vi "Get Errno Description.vi"(8 "error in":errorcluster, 11 "errnum":i32) -> (0 "error out":errorcluster, 3 "Description":string)   [LabVIEW 2018, in "PCANBasic.lvlib" / "epoll.lvclass"]
uses:
  epoll.lvclass
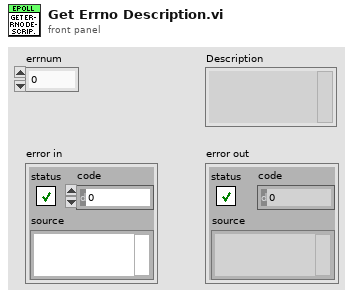
[diagram p1: front panel]
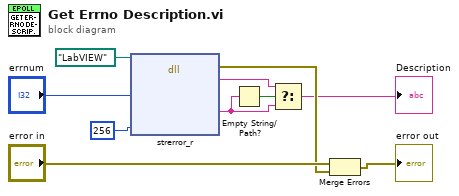
[diagram p0: block diagram]
diagram:
  n1 = dll-call lib="LabVIEW" fn="strerror_r"(path in=path "LabVIEW", "errnum"="errnum", "string_len"=256) -> (error out=w4:errorcluster, "return"=w6:string, "string"=w7:string)  [unwired: 5 in, 1 out]
  n2 = Empty String/Path?(string/path=w7) -> (empty?=w8:bool)
  n3 = Select(t=w6, s=w8, f=w7) -> (s? t:f=→"Description":string)
  n4 = Merge Errors("error in", w4) -> (→"error out":errorcluster)
